vi "IPS-Control.vi"(1 "Frage":string="A0", 2 "address string":string="25") -> (0 "Antwort":string="A\r")   [LabVIEW 2009]
panel:
  out "error out":errorcluster
  in  "error in (no error)":errorcluster
  in  "IPS Commands":string="C0   Local & Locked\nC3  Remote & Unlocked\n\nA0  Hold\nA1  To Set Point\nA2 To Zero\n\nH0 Switch Heater OFF\nH1 Switch Heater ON\n\nJnn Set Target Field\n\nTnn Set Field Sweep Rate\n\n\n\n"
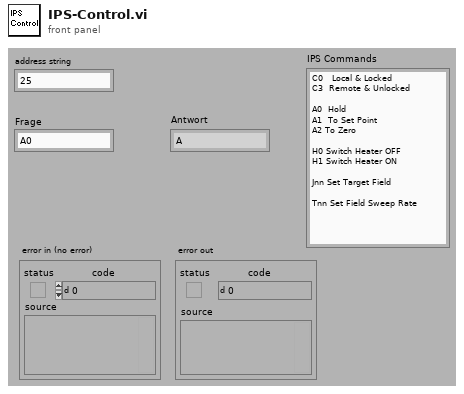
[diagram p1: front panel]
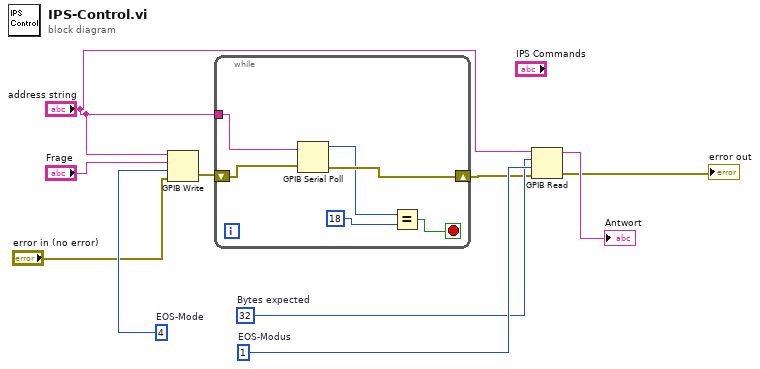
[diagram p0: block diagram]
diagram:
  w10 = 1  # EOS-Modus
  w9 = 32  # Bytes expected
  w8 = 4  # EOS-Mode
  n1 = GPIB Write(0:"address string", 1:"Frage", 2:w8, 3:"error in (no error)") -> (6:w4:errorcluster)  [unwired: 1 in, 1 out]
  n2 = while {
    shift-right: [w15] -> w3
    shift-left: w4 -> [w16]
    tunnel: "address string" -> [w14]
    stop <- w13 stop-if-true
    n3 = GPIB Serial Poll(0:w14, 1:w16) -> (2:w11:i16, 4:w15:errorcluster)  [unwired: 1 out]
    n4 = Equal?(x=w11, y=18) -> (x = y?=w13:bool)
  }
  n5 = GPIB Read(0:"address string", 1:w9, 2:w10, 3:w3) -> (5:→"Antwort":string, 7:→"error out":errorcluster)  [unwired: 1 in, 1 out]
